vi "settings-recall.vi"() -> (0 "error out":errorcluster, 3 "COM port":string, 5 "found?":bool)   [LabVIEW 2024]
uses:
  <vilib>/Utility/config.llb/Read Key (String).vi
  <vilib>/Utility/config.llb/NI_LVConfig.lvlib
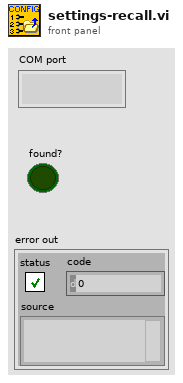
[diagram p1: front panel]
types:
  T1 = typedef "NI_LVConfig.lvlib/Config Data RefNum.ctl" = refnum<k1>
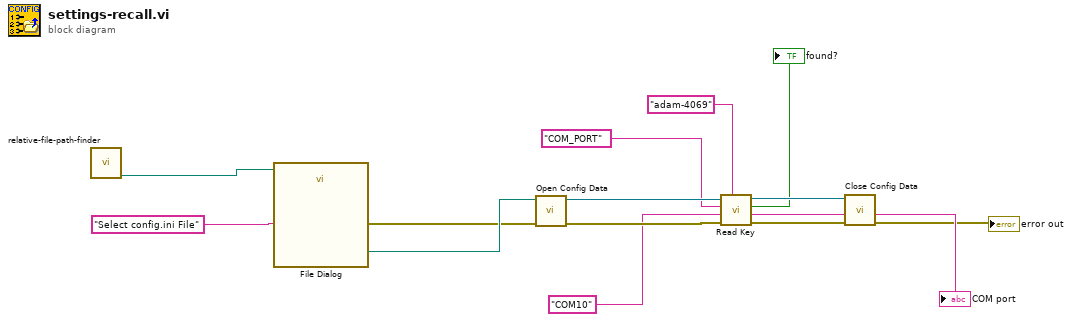
[diagram p0: block diagram]
diagram:
  n1 = call "relative-file-path-finder.vi"() -> ("Config File"=w3:path)  [unwired: 11 in]
  n2 = call "File Dialog"("start path"=w3, "prompt"="Select config.ini File") -> ("selected path"=w13:path, "error out"=w12:errorcluster)  [unwired: 10 in, 2 out]
  n3 = call <vilib>:"Open Config Data.vi"("error in (no error)"=w12, "configuration file path"=w13) -> ("error out"=w11:errorcluster, "refnum"=w10:T1)  [unwired: 7 in, 1 out]
  n4 = call-poly <vilib>:"Read Key.vi"("section"="adam-4069", "error in (no error)"=w11, "default value"="COM10", "key"="COM_PORT", "refnum"=w10) -> ("error out"=w5:errorcluster, "value"=→"COM port":string, "found?"=→"found?":bool, "refnum out"=w7:T1)  [unwired: 3 in]
  n5 = call <vilib>:"Close Config Data.vi"("error in (no error)"=w5, "refnum"=w7) -> ("error out"=→"error out":errorcluster)  [unwired: 8 in, 1 out]
